vi "Untitled 1.vi"() -> ()   [LabVIEW 2016]
panel:
  out "Waveform Chart":dbl(graph)
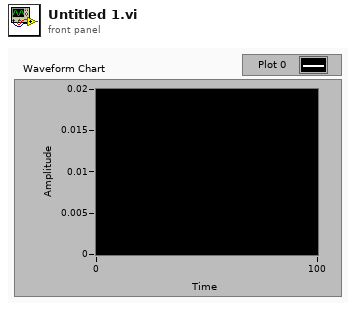
[diagram p1: front panel]
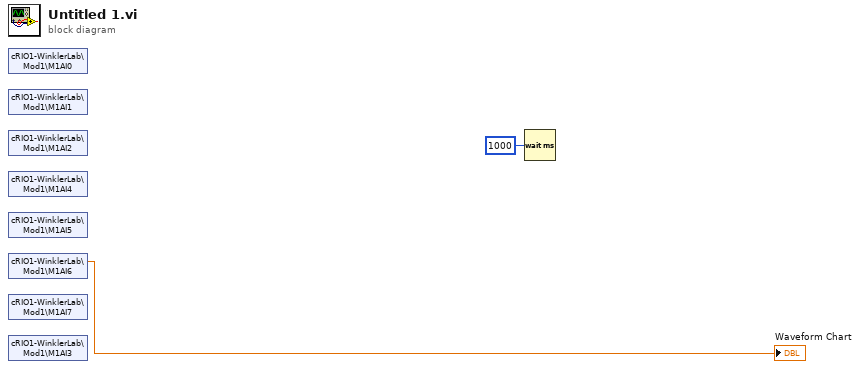
[diagram p0: block diagram]
diagram:
  n1 = shared-variable "cRIO1-WinklerLab\\Mod1\\M1AI0"() -> ()  [unwired: 1 in, 2 out]
  n2 = shared-variable "cRIO1-WinklerLab\\Mod1\\M1AI1"() -> ()  [unwired: 1 in, 2 out]
  n3 = shared-variable "cRIO1-WinklerLab\\Mod1\\M1AI2"() -> ()  [unwired: 1 in, 2 out]
  n4 = shared-variable "cRIO1-WinklerLab\\Mod1\\M1AI4"() -> ()  [unwired: 1 in, 2 out]
  n5 = shared-variable "cRIO1-WinklerLab\\Mod1\\M1AI5"() -> ()  [unwired: 1 in, 2 out]
  n6 = shared-variable "cRIO1-WinklerLab\\Mod1\\M1AI6"() -> (→"Waveform Chart":dbl)  [unwired: 1 in, 1 out]
  n7 = shared-variable "cRIO1-WinklerLab\\Mod1\\M1AI7"() -> ()  [unwired: 1 in, 2 out]
  n8 = shared-variable "cRIO1-WinklerLab\\Mod1\\M1AI3"() -> ()  [unwired: 1 in, 2 out]
  n9 = Wait (ms)(milliseconds to wait=u32 1000) -> ()  [unwired: 1 out]
